vi "Handle.vi"(7 "Event in":refnum<class "Event.lvclass">, 11 "Error State in":refnum<class "Error State.lvclass">) -> (2 "Destroy?":bool, 5 "Event out":refnum<class "Event.lvclass">)   [LabVIEW 2021, in "jettl.lvlib" / "Base Event.lvlib" / "State.lvlib" / "Error State.lvclass"]
uses:
  Error State.lvclass
  Event/Event.lvclass
  Error State.lvclass/Error State.ctl
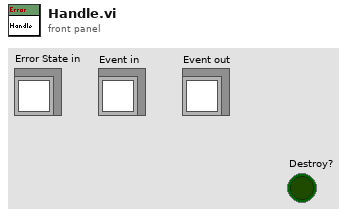
[diagram p1: front panel]
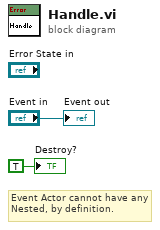
[diagram p0: block diagram]
diagram:
  # "Event Actor cannot have any Nested, by definition."
  "Destroy?" <- TRUE ("Destroy?")
  "Event out" <- "Event in"
